vi "SelectCam.vi"(8 "error in (no error)":errorcluster, 10 "Cam Session":string, 11 "Vision in":refnum<class "Vision.lvclass">) -> (0 "error out":errorcluster, 3 "Vision out":refnum<class "Vision.lvclass">)   [LabVIEW 2021, in "Vision.lvlib" / "Vision.lvclass"]
uses:
  Vision.lvclass
  Vision.lvclass/Vision.ctl
  <vilib>/userdefined/High Color/IMAQdx.ctl
  <vilib>/vision/driver/NI_Vision_Acquisition_Software.lvlib
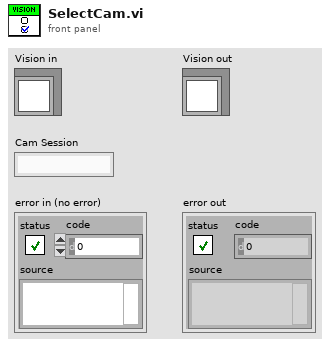
[diagram p1: front panel]
types:
  T1 = typedef "IMAQdx.ctl" = refnum<k21>
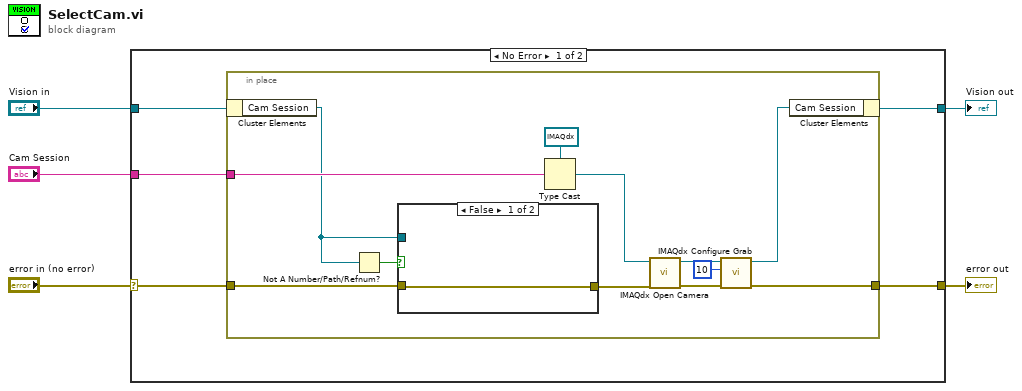
[diagram p0: block diagram]
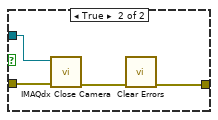
[diagram p2: hidden frame]
diagram:
  n1 = case shown="No Error" "error in (no error)" {
    selector: "error in (no error)" -> [w10 w29]
    tunnel: [w9 w29] -> w4
    tunnel: [w7 w28] -> w2
    tunnel: "Vision in" -> [w8 w28]
    tunnel: "Cam Session" -> [w6 _]
    frame No Error {
      n2 = in-place {
        in-place-border: w10 -> [w14]
        in-place-border: [w15] -> w9
        in-place-border: w6 -> [w21]
        n3 = in-place-cluster #1(w8) -> ("Cam Session"=w13:T1)
        n4 = Not A Number/Path/Refnum?(number/path/refnum=w13) -> (NaN/Path/Refnum?=w11:bool)
        n5 = case shown="False" w11 {
          tunnel: w14 -> [w23 w27]
          tunnel: w13 -> [_ w26]
          tunnel: [w23 w24] -> w12
          frame False {
          }
          frame True {
            n6 = call <vilib>:"IMAQdx Close Camera.vi"("error in"=w27, "Session In"=w26) -> ("error out"=w25:errorcluster)  [unwired: 9 in]
            n7 = call <vilib>:"Clear Errors.vi"("error in (no error)"=w25) -> ("error out"=w24:errorcluster)  [unwired: 5 in, 1 out]
          }
        }
        n8 = Type Cast(type=T1 refnum ("Cam Session"), x=w21) -> (*(type *) &x=w20:T1)
        n9 = call <vilib>:"IMAQdx Open Camera.vi"("error in"=w12, "Session In"=w20) -> ("error out"=w17:errorcluster, "Session Out"=w19:T1)  [unwired: 8 in]
        n10 = call <vilib>:"IMAQdx Configure Grab.vi"("error in"=w17, "Number of Buffers"=u32 10, "Session In"=w19) -> ("error out"=w15:errorcluster, "Session Out"=w16:T1)  [unwired: 7 in]
        n11 = in-place-cluster #1("Cam Session"=w16) -> (w7:refnum<class "Vision.lvclass">)
      }
    }
    frame Error {
    }
  }
  "error out" <- w4
  "Vision out" <- w2
